vi "SI101.vi"(0 "3 JEC10 CT001A XQ01":dbl, 1 "3 JEC20 CT001A XQ01":dbl, 2 "3 JEC30 CT001A XQ01":dbl, 3 "3 JEC40 CT001A XQ01":dbl, 4 "3 JEC10 CT001B XQ01":dbl, 5 "3 JEC20 CT001B XQ01":dbl, 6 "3 JEC30 CT001B XQ01":dbl, 7 "3 JEC40 CT001B XQ01":dbl, 8 "SI101_AverageReactorCoolantTemperature.lvclass":refnum<class "SI101.lvclass">, 9 "error in":errorcluster) -> (18 "SI101_AverageReactorCoolantTemperature.lvclass out":refnum<class "SI101.lvclass">, 19 "error out":errorcluster, 22 "ACT D-Comp":dbl, 23 "ACT 2ND MAX LIM":dbl, 24 "ACT 2nd Ctrl":dbl)   [LabVIEW 2022 SP3, in "SI101.lvclass"]
uses:
  SI101.lvclass
  SI101.lvclass/SI101.ctl
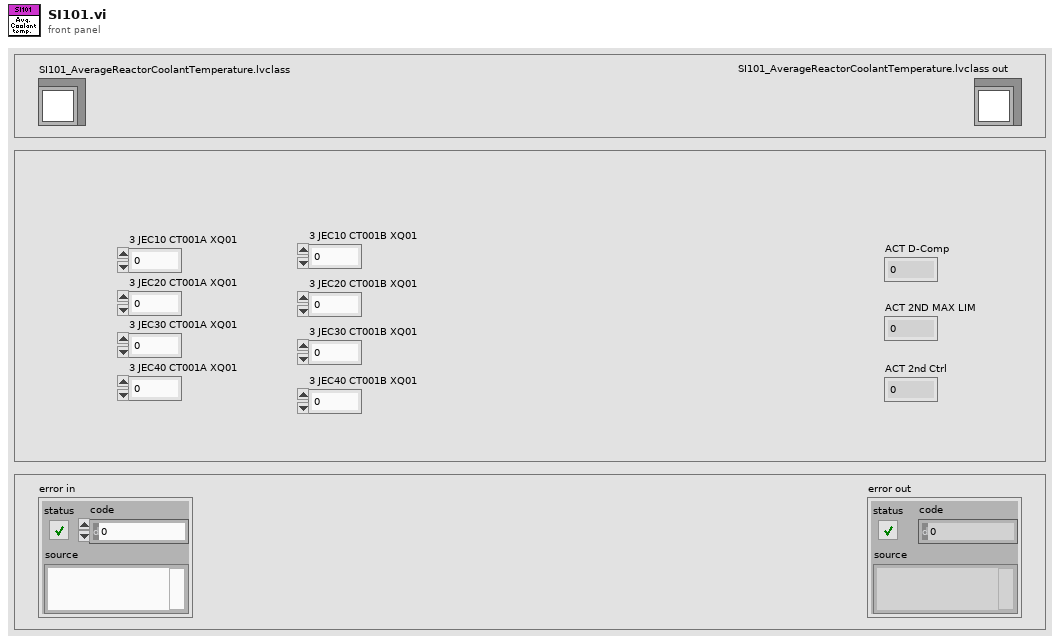
[diagram p1: front panel]
types:
  T1 = cluster{"JEC10CT001A":dbl, "JEC20CT001A":dbl, "JEC30CT001A":dbl, "JEC40CT001A":dbl}
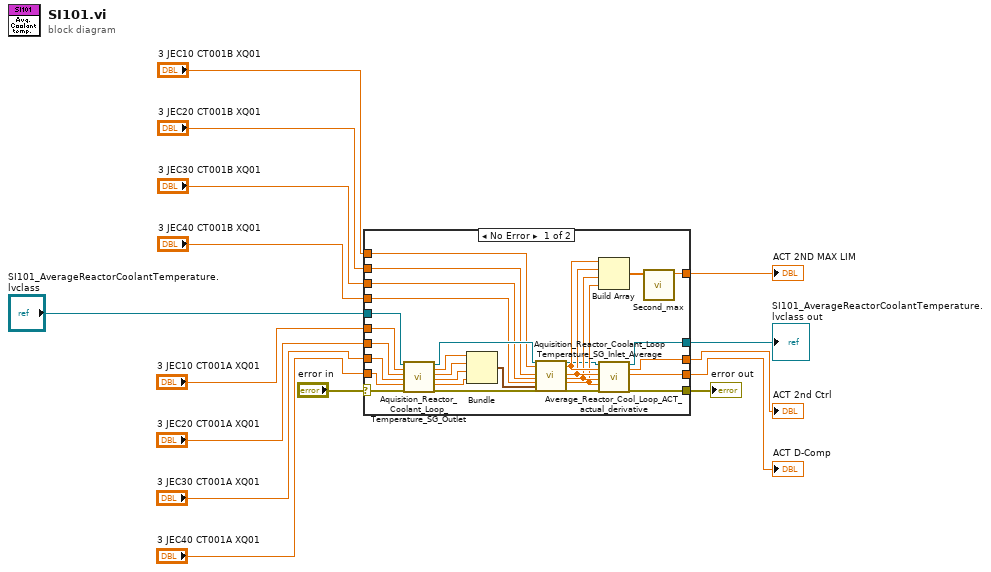
[diagram p0: block diagram]
diagram:
  n1 = case shown="No Error" "error in" {
    selector: "error in" -> [w44 w46]
    tunnel: "SI101_AverageReactorCoolantTemperature.lvclass" -> [w43 w45]
    tunnel: [w39 _] -> w13
    tunnel: [w34 _] -> w12
    tunnel: [w33 _] -> w11
    tunnel: [w30 w46] -> w10
    tunnel: [w29 w45] -> w9
    tunnel: "3 JEC10 CT001A XQ01" -> [w28 _]
    tunnel: "3 JEC20 CT001A XQ01" -> [w27 _]
    tunnel: "3 JEC30 CT001A XQ01" -> [w26 _]
    tunnel: "3 JEC40 CT001A XQ01" -> [w25 _]
    tunnel: "3 JEC10 CT001B XQ01" -> [w19 _]
    tunnel: "3 JEC20 CT001B XQ01" -> [w18 _]
    tunnel: "3 JEC30 CT001B XQ01" -> [w17 _]
    tunnel: "3 JEC40 CT001B XQ01" -> [w16 _]
    frame No Error {
      n2 = call "Aquisition_Reactor_Coolant_Loop_Temperature_SG_Outlet.vi"("SI101_AverageReactorCoolantTemperature.lvclass"=w43, "3 JEC10 CT001A XQ01"=w28, "3 JEC20 CT001A XQ01"=w27, "3 JEC30 CT001A XQ01"=w26, "3 JEC40 CT001A XQ01"=w25, "error in (no error)"=w44) -> ("SI101_AverageReactorCoolantTemperature.lvclass out"=w41:refnum<class "SI101.lvclass">, "JEC10CT001A"=w24:dbl, "JEC20CT001A"=w23:dbl, "JEC30CT001A"=w22:dbl, "JEC40CT001A"=w21:dbl, "error IO"=w42:errorcluster)  [unwired: 8 in]
      n3 = Bundle("JEC10CT001A"=w24, "JEC20CT001A"=w23, "JEC30CT001A"=w22, "JEC40CT001A"=w21) -> (w20:T1)  [unwired: 1 in]
      n4 = call "Aquisition_Reactor_Coolant_Loop Temperature_SG_Inlet_Average.vi"("SI101_AverageReactorCoolantTemperature.lvclass"=w41, "3 JEC10 CT001B XQ01"=w19, "3 JEC20 CT001B XQ01"=w18, "3 JEC30 CT001B XQ01"=w17, "3 JEC40 CT001B XQ01"=w16, "SG Outlet"=w20, "error in (no error)"=w42) -> ("SI101_AverageReactorCoolantTemperature.lvclass out"=w32:refnum<class "SI101.lvclass">, "ACT Loop 1"=w38:dbl, "ACT Loop 2"=w37:dbl, "ACT loop 3"=w36:dbl, "ACT loop 4"=w35:dbl, "error IO"=w31:errorcluster)  [unwired: 15 in]
      n5 = Build Array(w38, w37, w36, w35) -> (w40:dbl[])
      n6 = call "Average_Reactor_Cool_Loop_ACT_actual_derivative.vi"("SI101_AverageReactorCoolantTemperature.lvclass"=w32, "ACT Loop1"=w38, "ACT Loop2"=w37, "ACT Loop3"=w36, "ACT Loop4"=w35, "error in (no error)"=w31) -> ("SI101_AverageReactorCoolantTemperature.lvclass out"=w29:refnum<class "SI101.lvclass">, "ACT 2nd Ctrl"=w33:dbl, "ACT D-Comp"=w34:dbl, "error IO"=w30:errorcluster)  [unwired: 10 in]
      n7 = call "Second_max.vi"("Array"=w40) -> ("AP3"=w39:dbl)  [unwired: 10 in]
    }
    frame Error {
    }
  }
  "ACT 2ND MAX LIM" <- w13
  "ACT D-Comp" <- w12
  "ACT 2nd Ctrl" <- w11
  "error out" <- w10
  "SI101_AverageReactorCoolantTemperature.lvclass out" <- w9
